vi "Read position Remote.vi"(8 "error in (no error)":errorcluster, 11 "GameEl in":refnum<class "GameEl.lvclass">) -> (0 "error out":errorcluster, 3 "position":cluster{"x":dbl, "y":dbl}[](array[cluster]))   [LabVIEW 2021, in "GameEl.lvclass"]
uses:
  GameEl.lvclass
  GameEl.lvclass/GameEl.ctl
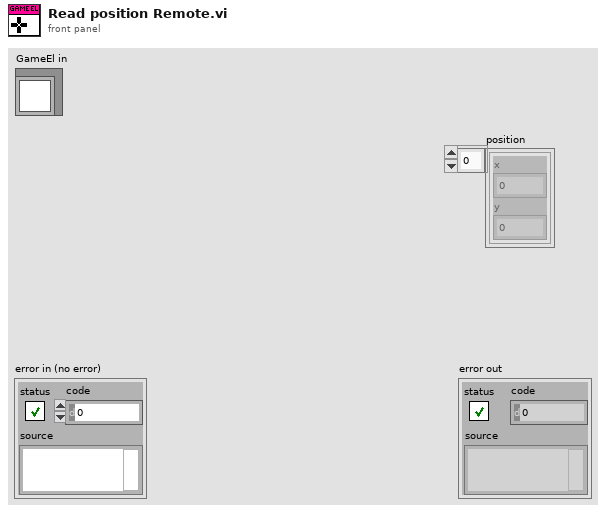
[diagram p1: front panel]
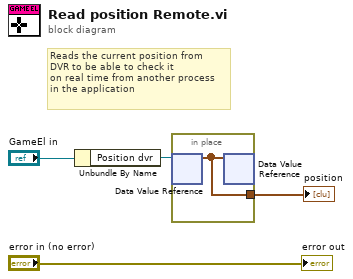
[diagram p0: block diagram]
diagram:
  # "Reads the current position from \nDVR to be able to check it \non real time from another process\nin the application"
  n1 = Unbundle By Name("GameEl in") -> ("Position dvr"=w2:refnum<data-value>)
  n2 = in-place {
    in-place-border: [w5] -> w1
    n3 = in-place-dvr #1(w2) -> (w5:cluster{"x":dbl, "y":dbl}[])  [unwired: 1 out]
    n4 = in-place-dvr #1(w5) -> ()  [unwired: 2 out]
  }
  "position" <- w1
  "error out" <- "error in (no error)"
